vi "getPoints.vi"(0 "reference":refnum<class "CallEdge.lvclass">, 5 "error in (no error)":errorcluster) -> (14 "reference out":refnum<class "CallEdge.lvclass">, 15 "points":T1[](array[typedef]) {"y" format="%.2f"; "x" format="%.2f"}, 19 "error out":errorcluster)   [LabVIEW 2012, in "CallEdge.lvclass"]
doc: "public ArrayList getPoints()"
uses:
  <resource>/Framework/Providers/Open_GDS/UML/CallEdge_class/CallEdge.lvclass
  <resource>/Framework/Providers/Open_GDS/UML/General/Point/Point Point2D.ctl
  <resource>/Framework/Providers/Open_GDS/UML/CallNode_class/CallNode.lvclass
  <resource>/Framework/Providers/Open_GDS/UML/AbstractNode_class/AbstractNode.lvclass
  <resource>/Framework/Providers/Open_GDS/UML/Direction_class/Direction.lvclass
  <resource>/Framework/Providers/Open_GDS/UML/AbstractEdge_class/AbstractEdge.lvclass
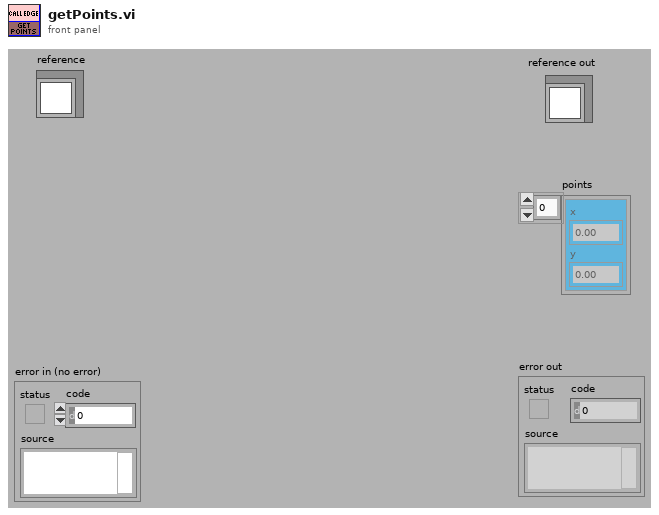
[diagram p1: front panel]
types:
  T1 = typedef "Point Point2D.ctl" = cluster{"x":dbl, "y":dbl}
  T2 = typedef "AbstractEdge.lvclass/ObjectAttributes.ctl" = cluster{"start":refnum<class "AbstractNode.lvclass">, "end":refnum<class "AbstractNode.lvclass">}
  T3 = typedef "Rectangle Rectangle2D.ctl" = cluster{"x":dbl, "y":dbl, "width":dbl, "height":dbl}
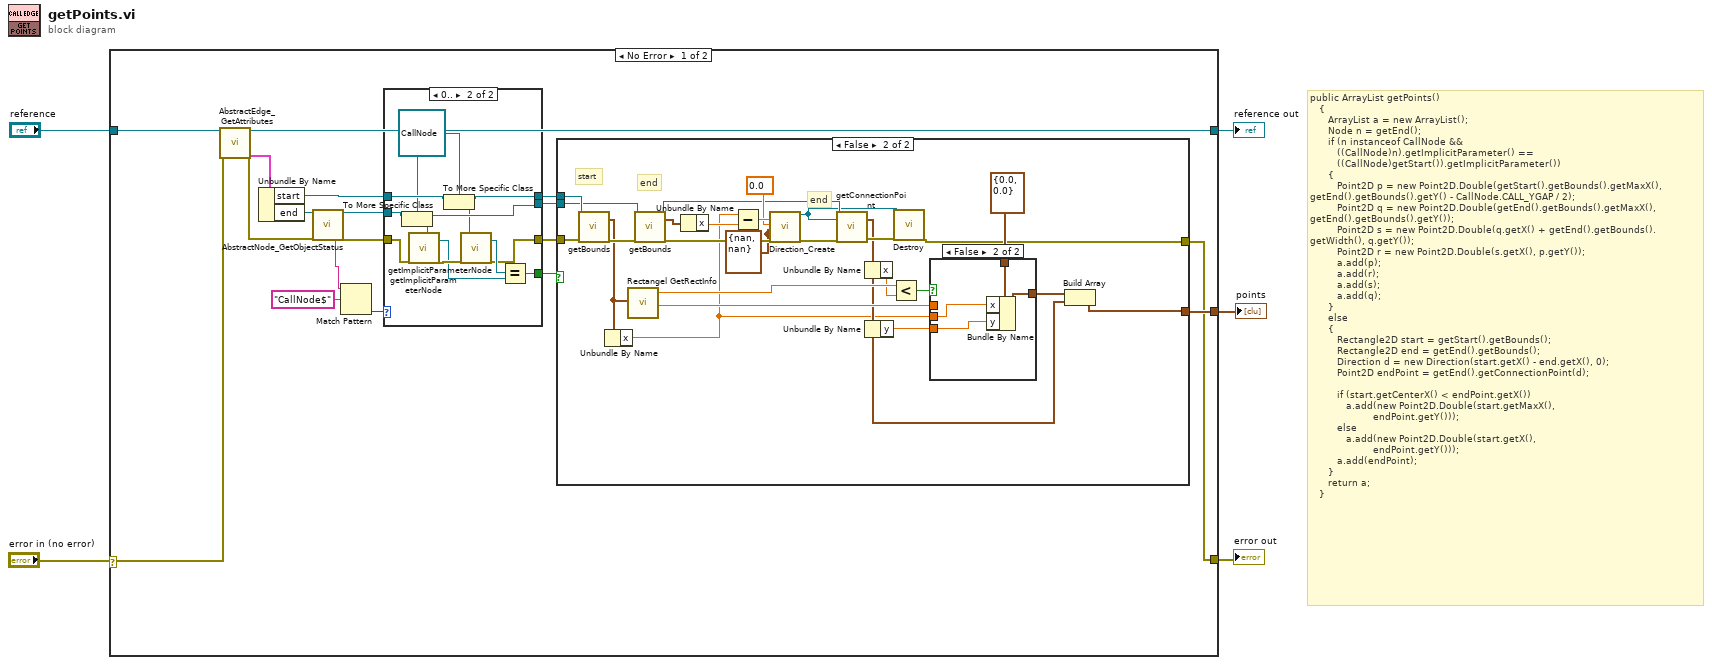
[diagram p0: block diagram]
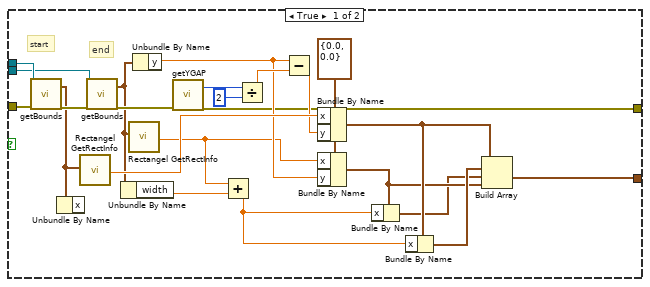
[diagram p2: hidden frame]
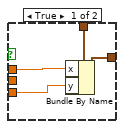
[diagram p3: hidden frame]
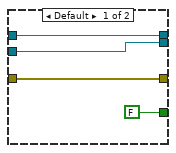
[diagram p4: hidden frame]
diagram:
  # "public ArrayList getPoints()\n   {\n      ArrayList a = new ArrayList();\n      Node n = getEnd();\n      if (n instanceof CallNode &&\n         ((CallNode)n).getImplicitParameter() ==\n         ((CallNode)getStart()).getImplicitParameter())\n      {\n         Point2D p = new Point2D.Double(getStart().getBounds().getMaxX(), getEnd().getBounds().getY() - CallNode.CALL_YGAP / 2);\n         Point2D q = new Point2D.Double(getEnd().getBounds().getMaxX(), getEnd().getBounds().getY());\n         Point2D s = new Point2D.Double(q.getX() + getEnd().getBounds().getWidth(), q.getY());\n         Point2D r = new Point2D.Double(s.getX(), p.getY());\n         a.add(p);\n         a.add(r);\n         a.add(s);\n         a.add(q);\n      }\n      else\n      {\n         Rectangle2D start = getStart().getBounds();\n         Rectangle2D end = getEnd().getBounds();\n         Direction d = new Direction(start.getX() - end.getX(), 0);\n         Point2D endPoint = getEnd().getConnectionPoint(d);\n         \n         if (start.getCenterX() < endPoint.getX())\n            a.add(new Point2D.Double(start.getMaxX(),\n                     endPoint.getY()));\n         else\n            a.add(new Point2D.Double(start.getX(),\n                     endPoint.getY()));\n         a.add(endPoint);\n      }\n      return a;\n   }"
  n1 = case shown="No Error" "error in (no error)" {
    selector: "error in (no error)" -> [w21 w96]
    tunnel: "reference" -> [w23 w97]
    tunnel: [w19 w96] -> w4
    tunnel: [w22 w97] -> w3
    tunnel: [w20 _] -> w1
    frame No Error {
      n2 = call <resource>:"AbstractEdge_GetAttributes.vi"("reference in"=w23, "error in (no error)"=w21) -> ("reference out"=w22:refnum<class "CallEdge.lvclass">, "Data"=w7:T2, "error out"=w12:errorcluster)  [unwired: 14 in, 1 out]
      n3 = Unbundle By Name(w7) -> ("start"=w14:refnum<class "AbstractNode.lvclass">, "end"=w18:refnum<class "AbstractNode.lvclass">)
      n4 = call <resource>:"AbstractNode_GetObjectStatus.vi"("reference in"=w18, "error in (no error)"=w12) -> ("Class name"=w6:string, "reference out"=w15:refnum<class "AbstractNode.lvclass">, "error out"=w13:errorcluster)  [unwired: 15 out]
      n5 = Match Pattern(string=w6, regular expression="CallNode$") -> (offset past match=w16:i32)  [unwired: 4 out]
      n6 = case shown="0.." w16 {
        tunnel: w15 -> [w81 w89]
        tunnel: w14 -> [w82 w88]
        tunnel: w13 -> [w83 w94]
        tunnel: [FALSE w92] -> w11
        tunnel: [w83 w91] -> w10
        tunnel: [w82 w85] -> w9
        tunnel: [w81 w87] -> w8
        frame Default {
        }
        frame 0.. {
          w86 = refnum<class "CallNode.lvclass"> refnum ("reference")
          n7 = To More Specific Class(target class=w86, reference=w89) -> (specific class reference=w87:refnum<class "CallNode.lvclass">)  [unwired: 1 in, 1 out]
          n8 = call-dynamic "getImplicitParameterNode.vi"("reference"=w87, "error in (no error)"=w94) -> ("objectCallNodeRef"=w90:refnum<class "AbstractNode.lvclass">, "error out"=w93:errorcluster)  [unwired: 15 in, 1 out]
          n9 = To More Specific Class(target class=w86, reference=w88) -> (specific class reference=w85:refnum<class "CallNode.lvclass">)  [unwired: 1 in, 1 out]
          n10 = call-dynamic "getImplicitParameterNode.vi"("reference"=w85, "error in (no error)"=w93) -> ("objectCallNodeRef"=w95:refnum<class "AbstractNode.lvclass">, "error out"=w91:errorcluster)  [unwired: 15 in, 1 out]
          n11 = Equal?(x=w95, y=w90) -> (x = y?=w92:bool)
        }
      }
      n12 = case shown="False" w11 {
        tunnel: w10 -> [w44 w70]
        tunnel: [w46 w72] -> w20
        tunnel: w9 -> [w42 w68]
        tunnel: w8 -> [w41 w67]
        tunnel: [w27 w48] -> w19
        frame True {
          w45 = T1 {"x"=0.0, "y"=0.0} ("point2D")
          # "end"
          # "start"
          n13 = call-dynamic "getBounds.vi"("reference"=w42, "error in (no error)"=w44) -> ("bounds"=w39:T3, "error out"=w43:errorcluster)  [unwired: 15 in, 1 out]
          n14 = Unbundle By Name(w39) -> ()  [unwired: 1 out]
          n15 = call <resource>:"Rectangel GetRectInfo.vi"("bounds"=w39) -> ("maxX"=w40:dbl)  [unwired: 1 in, 17 out]
          n16 = call-dynamic "getBounds.vi"("reference"=w41, "error in (no error)"=w43) -> ("bounds"=w31:T3, "error out"=w38:errorcluster)  [unwired: 15 in, 1 out]
          n17 = Unbundle By Name(w31) -> ("width"=w30:dbl)
          n18 = call <resource>:"Rectangel GetRectInfo.vi"("bounds"=w31) -> ("maxX"=w29:dbl)  [unwired: 1 in, 17 out]
          n19 = Unbundle By Name(w31) -> ("y"=w33:dbl)
          n20 = call <resource>:"getYGAP.vi"("error in (no error)"=w38) -> ("CALL_YGAP"=w37:i32, "error out"=w27:errorcluster)  [unwired: 17 out]
          n21 = Add(x=w29, y=w30) -> (x+y=w28:dbl)
          n22 = Divide(x=w37, y=2) -> (x/y=w35:dbl)
          n23 = Subtract(x=w33, y=w35) -> (x-y=w34:dbl)
          n24 = Bundle By Name(cluster=w45, "x"=w40, "y"=w34) -> (w32:T1)
          n25 = Bundle By Name(cluster=w45, "x"=w29, "y"=w33) -> (w25:T1)
          n26 = Bundle By Name(cluster=w25, "x"=w28) -> (w24:T1)
          n27 = Bundle By Name(cluster=w32, "x"=w28) -> (w26:T1)
          n28 = Build Array(w32, w26, w24, w25) -> (w46:T1[])
        }
        frame False {
          w47 = T1 {"x"=nan, "y"=nan} ("p1")
          # "end"
          # "end"
          # "start"
          n29 = call-dynamic "getBounds.vi"("reference"=w68, "error in (no error)"=w70) -> ("bounds"=w66:T3, "error out"=w69:errorcluster)  [unwired: 15 in, 1 out]
          n30 = Unbundle By Name(w66) -> ("x"=w49:dbl)
          n31 = call <resource>:"Rectangel GetRectInfo.vi"("bounds"=w66) -> ("centerX"=w56:dbl, "maxX"=w52:dbl)  [unwired: 1 in, 16 out]
          n32 = call-dynamic "getBounds.vi"("reference"=w67, "error in (no error)"=w69) -> ("reference out"=w59:refnum<class "AbstractNode.lvclass">, "bounds"=w65:T3, "error out"=w64:errorcluster)  [unwired: 15 in]
          n33 = Unbundle By Name(w65) -> ("x"=w62:dbl)
          n34 = Subtract(x=w49, y=w62) -> (x-y=w63:dbl)
          n35 = call <resource>:"Direction_Create.vi"("dx"=w63, "dy"=0.0, "p1"=w47, "p2"=w47, "error in (no error)"=w64) -> ("reference out"=w57:refnum<class "Direction.lvclass">, "error out"=w60:errorcluster)  [unwired: 13 in]
          n36 = call-dynamic "getConnectionPoint.vi"("reference"=w59, "direction"=w57, "error in (no error)"=w60) -> ("point2D"=w51:T1, "error out"=w58:errorcluster)  [unwired: 14 in, 1 out]
          n37 = Unbundle By Name(w51) -> ("x"=w55:dbl)
          n38 = Unbundle By Name(w51) -> ("y"=w50:dbl)
          n39 = Less?(x=w56, y=w55) -> (x < y?=w54:bool)
          n40 = call-dynamic "Destroy.vi"("reference"=w57, "error in (no error)"=w58) -> ("error out"=w48:errorcluster)  [unwired: 17 in]
          n41 = case shown="False" w54 {
            tunnel: T1 {"x"=0.0, "y"=0.0} ("point2D") -> [w76 w80]
            tunnel: [w75 w79] -> w53
            tunnel: w52 -> [w74 _]
            tunnel: w50 -> [w73 w78]
            tunnel: w49 -> [_ w77]
            frame True {
              n42 = Bundle By Name(cluster=w76, "x"=w74, "y"=w73) -> (w75:T1)
            }
            frame False {
              n43 = Bundle By Name(cluster=w80, "x"=w77, "y"=w78) -> (w79:T1)
            }
          }
          n44 = Build Array(w53, w51) -> (w72:T1[])
        }
      }
    }
    frame Error {
    }
  }
  "reference out" <- w3
  "error out" <- w4
  "points" <- w1
